vi "GM Count.vi"(0 "QUIT":refnum<vi>, 1 "Scan in Progress":refnum<vi>, 2 "Measure":refnum<vi>, 3 "Error":refnum<vi>, 8 "Dwell Right":refnum<vi>, 10 "LLD Right":refnum<vi>, 12 "ULD Right":refnum<vi>, 14 "Counts Right":refnum<vi>) -> ()   [LabVIEW 2017]
uses:
  <vilib>/DAQmx/read.llb/DAQmx Read (Counter 1D U32 1Chan NSamp).vi
panel:
  out "Right Storage":dbl[](array[numeric])
  in  "GM Count":enum32{"Geiger-Muller Photodetectors", "Errors"}(tab)
  out "Average Right":dbl caption="Average Rate"
  in  "ULD Right":dbl caption="Upper Limit" max=12.0
  in  "Dwell Right 2":dbl=1.0 caption="Dwell" min=0.1
  in  "LLD Right":dbl caption="Lower Limit" max=12.0
  out "Counts Right 2":u32 caption="Counts"
  out "Rate Right":dbl caption="Count Rate"
  in  "Number of Rates\nto Average":u32=20 min=1
  out "Error":errorcluster
  # "Note that the Average Rate is found by simply averaging the last 'n' acquired count rates.  Therefore,\nit may not be an accurate measure of the real count rate in Hz if Dwell has recently been changed."
  # "Left"
  # "Right"
  # "s"
  # "V"
  # "Hz"
  # "V"
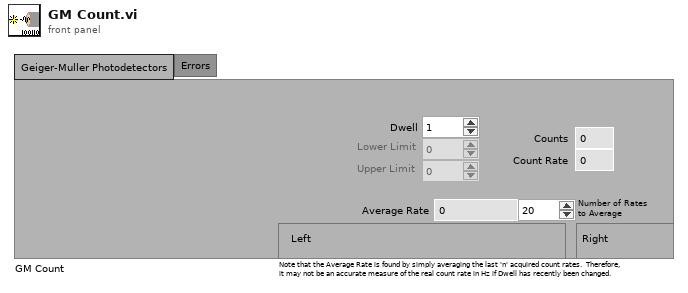
[diagram p1: front panel]
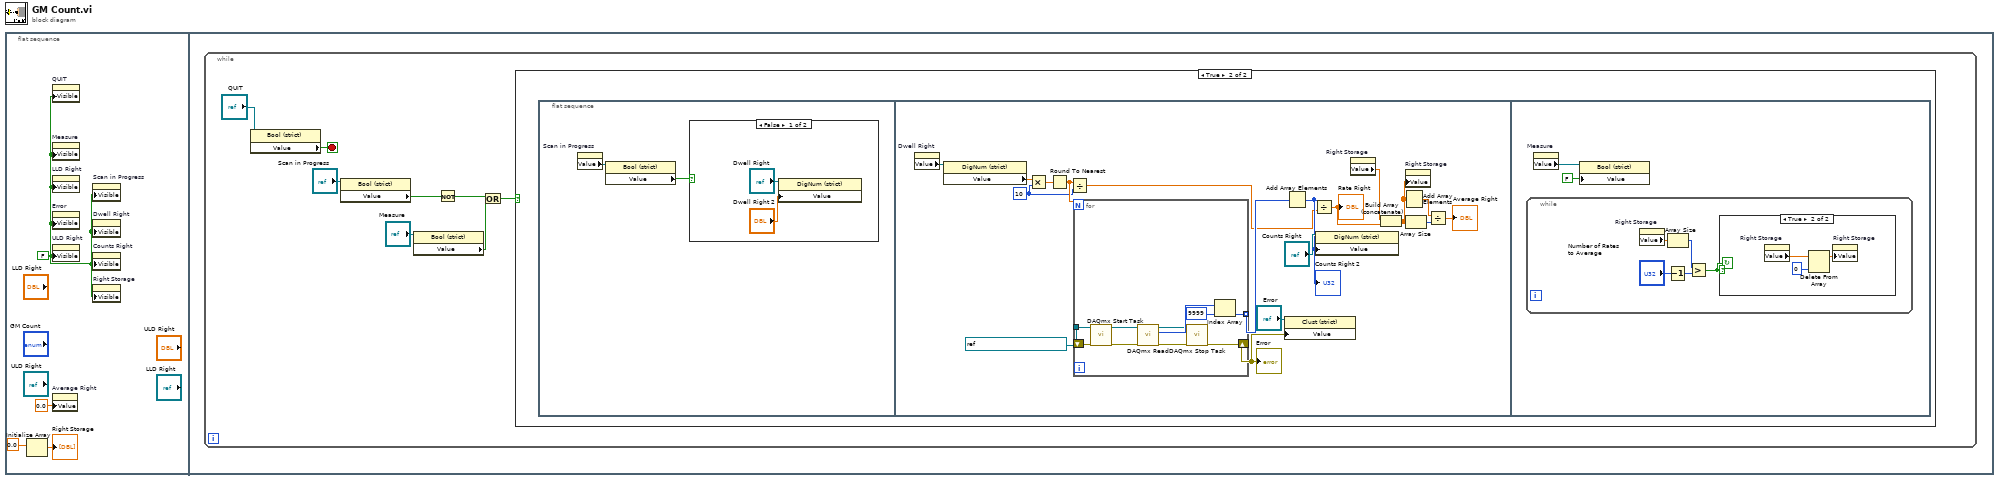
[diagram p0: block diagram]
diagram:
  n1 = flat-sequence {
    frame #0 {
      w1 = FALSE ("Visible")
      n2 = Initialize Array(0.0 ("element")) -> (→"Right Storage":dbl[])  [unwired: 1 in]
      n3 = property on="QUIT" class="LVObjRef (strict)"("Visible"=w1) -> ()  [unwired: 2 in, 2 out]
      n4 = property on="Measure" class="LVObjRef (strict)"("Visible"=w1) -> ()  [unwired: 2 in, 2 out]
      n5 = property on="LLD Right" class="LVObjRef (strict)"("Visible"=w1) -> ()  [unwired: 2 in, 2 out]
      n6 = property on="Error" class="LVObjRef (strict)"("Visible"=w1) -> ()  [unwired: 2 in, 2 out]
      n7 = property on="ULD Right" class="LVObjRef (strict)"("Visible"=w1) -> ()  [unwired: 2 in, 2 out]
      n8 = property on="Average Right" class="DigNum (strict)"("Value"=0.0 ("Average Right")) -> ()  [unwired: 2 in, 2 out]
      n9 = property on="Scan in Progress" class="LVObjRef (strict)"("Visible"=w1) -> ()  [unwired: 2 in, 2 out]
      n10 = property on="Dwell Right" class="LVObjRef (strict)"("Visible"=w1) -> ()  [unwired: 2 in, 2 out]
      n11 = property on="Counts Right" class="LVObjRef (strict)"("Visible"=w1) -> ()  [unwired: 2 in, 2 out]
      n12 = property on="Right Storage" class="Arr (strict)"("Visible"=w1) -> ()  [unwired: 2 in, 2 out]
    }
    frame #1 {
      n13 = while {
        stop <- w11 stop-if-true
        n14 = property on="Property Node" class="Bool (strict)"(reference="QUIT") -> ("Value"=w11:bool)  [unwired: 1 in, 2 out]
        n15 = property on="Property Node" class="Bool (strict)"(reference="Scan in Progress") -> ("Value"=w9:bool)  [unwired: 1 in, 2 out]
        n16 = property on="Property Node" class="Bool (strict)"(reference="Measure") -> ("Value"=w6:bool)  [unwired: 1 in, 2 out]
        n17 = Not(x=w9) -> (.not. x?=w8:bool)
        n18 = Or(x=w8, y=w6) -> (x .or. y?=w5:bool)
        n19 = case shown="True" w5 {
          frame False {
          }
          frame True {
            n20 = flat-sequence {
              frame #0 {
                n21 = property on="Scan in Progress" class="LVObjRef (strict)"() -> ("Value"=w14:refnum<vi>)  [unwired: 2 in, 2 out]
                n22 = property on="Property Node" class="Bool (strict)"(reference=w14) -> ("Value"=w13:bool)  [unwired: 1 in, 2 out]
                n23 = case shown="False" w13 {
                  frame False {
                    n24 = property on="Property Node" class="DigNum (strict)"(reference="Dwell Right", "Value"="Dwell Right 2") -> ()  [unwired: 1 in, 2 out]
                  }
                  frame True {
                  }
                }
              }
              frame #1 {
                w25 = 10 ("y")
                n25 = property on="Dwell Right" class="LVObjRef (strict)"() -> ("Value"=w23:refnum<vi>)  [unwired: 2 in, 2 out]
                n26 = property on="Property Node" class="DigNum (strict)"(reference=w23) -> ("Value"=w28:dbl)  [unwired: 1 in, 2 out]
                n27 = Multiply(x=w28, y=w25) -> (x*y=w27:dbl)
                n28 = Round To Nearest(number=w27) -> (nearest integer value=w26:dbl)
                n29 = Divide(x=w26, y=w25) -> (x/y=w24:dbl)
                n30 = for {
                  N: w26 -> [_]
                  tunnel: refnum<k21> "GM Count Pulses Right" ("task/channels in") -> [w44]
                  shift-right: [w36] -> w31
                  shift-left: _ -> [w43]
                  tunnel: [w38] -> w33 mode=indexing
                  n31 = call <vilib>:"DAQmx Start Task.vi"("task/channels in"=w44, "error in"=w43) -> ("task out"=w42:refnum<k21>, "error out"=w41:errorcluster)  [unwired: 12 in]
                  n32 = call-poly <vilib>:"DAQmx Read.vi"("task/channels in"=w42, "error in"=w41) -> ("task out"=w35:refnum<k21>, "data"=w40:u32[], "error out"=w37:errorcluster)  [unwired: 11 in]
                  n33 = call <vilib>:"DAQmx Stop Task.vi"("task/channels in"=w35, "error in"=w37) -> ("error out"=w36:errorcluster)  [unwired: 12 in, 1 out]
                  n34 = Index Array(array=w40, index=9999) -> (element=w38:u32)
                }
                "Error" <- w31
                n35 = property on="Property Node" class="Clust (strict)"(reference="Error", "Value"=w31) -> ()  [unwired: 1 in, 2 out]
                n36 = Add Array Elements(numeric array=w33) -> (sum=w29:u32)
                "Counts Right 2" <- w29
                n37 = Divide(x=w29, y=w24) -> (x/y=w21:dbl)
                "Rate Right" <- w21
                n38 = property on="Property Node" class="DigNum (strict)"(reference="Counts Right", "Value"=w29) -> ()  [unwired: 1 in, 2 out]
                n39 = property on="Right Storage" class="Arr (strict)"() -> ("Value"=w22:dbl[])  [unwired: 2 in, 2 out]
                n40 = Build Array (concatenate)(w22, w21) -> (w17:dbl[])
                n41 = Add Array Elements(numeric array=w17) -> (sum=w20:dbl)
                n42 = property on="Right Storage" class="Arr (strict)"("Value"=w17) -> ()  [unwired: 2 in, 2 out]
                n43 = Array Size(array=w17) -> (size(s)=w19:i32)
                n44 = Divide(x=w20, y=w19) -> (x/y=→"Average Right":dbl)
              }
              frame #2 {
                n45 = while {
                  stop <- w49 continue-if-true
                  n46 = property on="Right Storage" class="Arr (strict)"() -> ("Value"=w50:dbl[])  [unwired: 2 in, 2 out]
                  n47 = Decrement(x="Number of Rates\nto Average") -> (x-1=w48:u32)
                  n48 = Array Size(array=w50) -> (size(s)=w51:i32)
                  n49 = Greater?(x=w51, y=w48) -> (0:w49:bool)
                  n50 = case shown="True" w49 {
                    frame False {
                    }
                    frame True {
                      n51 = property on="Right Storage" class="Arr (strict)"() -> ("Value"=w54:dbl[])  [unwired: 2 in, 2 out]
                      n52 = Delete From Array(array=w54, index=0) -> (array with subset deleted=w52:dbl[])  [unwired: 1 in, 1 out]
                      n53 = property on="Right Storage" class="Arr (strict)"("Value"=w52) -> ()  [unwired: 2 in, 2 out]
                    }
                  }
                }
                n54 = property on="Measure" class="LVObjRef (strict)"() -> ("Value"=w46:refnum<vi>)  [unwired: 2 in, 2 out]
                n55 = property on="Property Node" class="Bool (strict)"(reference=w46, "Value"=FALSE) -> ()  [unwired: 1 in, 2 out]
              }
            }
          }
        }
      }
    }
  }
